vi "误差计算.vi"(6 "第几组":i32, 7 "选择?":bool[](array[boolean]), 8 "允许误差":dbl, 9 "模拟量量程范围":dbl, 10 "设定值_1":dbl, 11 "反馈值_1":dbl) -> (0 "字符串_误差_1":string, 2 "误差_1":dbl, 3 "合格_1?":bool)   [LabVIEW 2010]
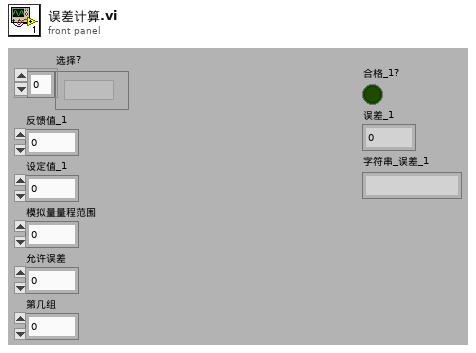
[diagram p1: front panel]
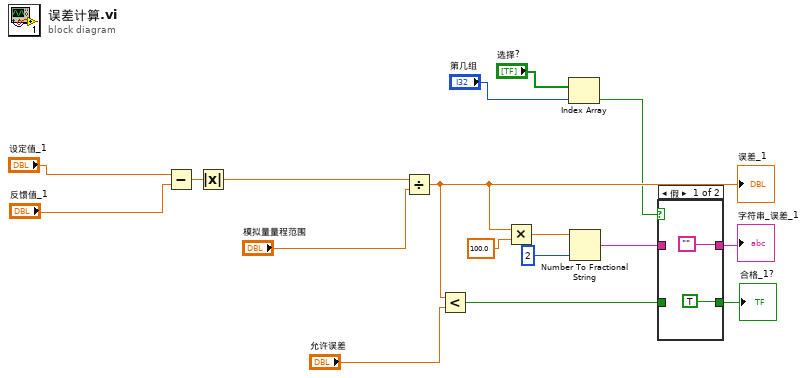
[diagram p0: block diagram]
diagram:
  n1 = Subtract(x="设定值_1", y="反馈值_1") -> (x-y=w17:dbl)
  n2 = Absolute Value(x=w17) -> (abs(x)=w15:dbl)
  n3 = Divide(x=w15, y="模拟量量程范围") -> (x/y=w11:dbl)
  "误差_1" <- w11
  n4 = Less?(x=w11, y="允许误差") -> (x < y?=w4:bool)
  n5 = Multiply(x=w11, y=100.0) -> (x*y=w12:dbl)
  n6 = Index Array(array="选择?", index="第几组") -> (element=w7:bool)
  n7 = Number To Fractional String(number=w12, precision (6)=i16 2 ("精度(6)")) -> (F-format string=w6:string)  [unwired: 2 in]
  n8 = case shown="假" w7 {
    tunnel: w6 -> [_ w21]
    tunnel: ["" w21] -> w5
    tunnel: w4 -> [_ w20]
    tunnel: [TRUE w20] -> w3
    frame False {
    }
    frame True {
    }
  }
  "合格_1?" <- w3
  "字符串_误差_1" <- w5
